vi "DataLib.unpack data.vi"(1 "dataIn":T1, 5 "error in (no error)":errorcluster) -> (15 "remainingData":T1, 16 "DAQDevice":string, 17 "Data Descriptor":T2, 18 "DAQDeviceData":T1, 19 "error out":errorcluster)   [LabVIEW 2014, in "DataLib.lvlib"]
doc: "Unpacks the data of each DAQ device. This routine can be used to unpack device data delivered by the EventBuilder class.\n\nComment: This routine is not intended to be used by end-users. End users should unpack data from an EventBuilder (or a DiscArchiver) using the methods \"unpack event data\" and \"unpack subevent data\" (\"unpack subevent data\")."
uses:
  DataLib.lvlib
  CS_Core/CSSystem/CoreDefs/CoreDefs.rawDataType.ctl
  CS_Core/BaseProcess/BaseProcess.descriptor string definition.ctl
  CS_Core/CSSystem/CoreLib/CoreLib.byte array 2 string.vi
  CS_Core/CSSystem/CoreLib/CoreLib.lvlib
  CS_Core/BaseProcess/BaseProcess.lvlib
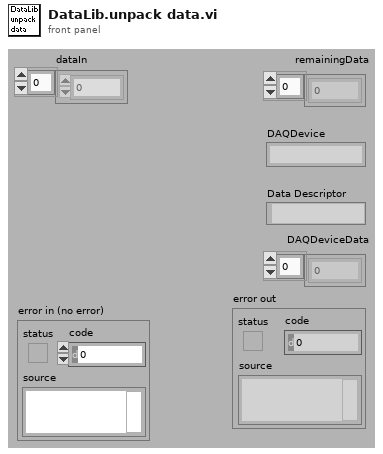
[diagram p1: front panel]
types:
  T1 = typedef "CoreDefs.rawDataType.ctl" = i8[]
  T2 = typedef "BaseProcess.lvlib/BaseProcess.descriptor string definition.ctl" = string
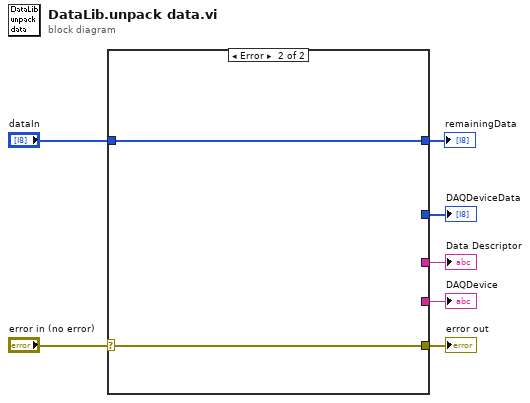
[diagram p0: block diagram]
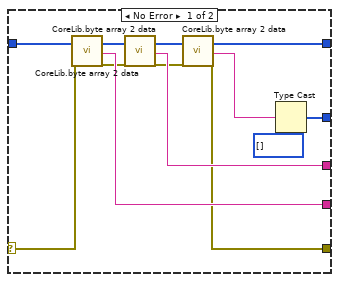
[diagram p2: hidden frame]
diagram:
  n1 = case shown="Error" "error in (no error)" {
    selector: "error in (no error)" -> [w15 w22]
    tunnel: "dataIn" -> [w20 w21]
    tunnel: [w18 _] -> w6
    tunnel: [w17 _] -> w5
    tunnel: [w9 _] -> w4
    tunnel: [w12 w22] -> w2
    tunnel: [w8 w21] -> w1
    frame No Error {
      n2 = call-poly "CoreLib.byte array 2 data.vi"("byteArray"=w20, "error in (no error)"=w15) -> ("byteArray out"=w19:T1, "string"=w18:string, "error out"=w16:errorcluster)  [unwired: 15 in]
      n3 = call-poly "CoreLib.byte array 2 data.vi"("byteArray"=w19, "error in (no error)"=w16) -> ("byteArray out"=w14:T1, "string"=w17:string, "error out"=w13:errorcluster)  [unwired: 15 in]
      n4 = call-poly "CoreLib.byte array 2 data.vi"("byteArray"=w14, "error in (no error)"=w13) -> ("byteArray out"=w8:T1, "string"=w11:string, "error out"=w12:errorcluster)  [unwired: 15 in]
      n5 = Type Cast(type=T1 [] ("Array"), x=w11) -> (*(type *) &x=w9:T1)
    }
    frame Error {
    }
  }
  "DAQDeviceData" <- w4
  "Data Descriptor" <- w5
  "DAQDevice" <- w6
  "error out" <- w2
  "remainingData" <- w1
